vi "main.vi"() -> ()   [LabVIEW 2011]
uses:
  tab1.ctl
  System.Windows.Forms
  usb webcam list.ctl
  <vilib>/Instr/_visa.llb/VISA Configure Serial Port (Instr).vi
  <vilib>/vision/NI_Vision_Development_Module.lvlib
  <vilib>/Utility/file.llb/Read From Spreadsheet File (string).vi
  <vilib>/Utility/file.llb/Write To Spreadsheet File (string).vi
panel:
  out "height less than 1cm(80pixels)":bool
  out "image features":T1
  out "Vertical Profile":sgl[](graph)
  in  "cam on":bool=TRUE
  out "Clipboard has an image?":bool
  in  "stop for camera":bool
  in  "Select options":T2(radio)=enum."Database testing"
  in  "Tab Control 2":T3(tab)
  in  "Show cyl list":bool
  out "cust list":string[](array[string])
  in  "select cust":string
  out "cyl list":string[](array[string])
  out "cust data":string[][](array[string])
  out "weightage Array":u8[][](array[numeric])
  out "read matrix":u8[][](array[numeric])
  out "correlation":u8[](array[numeric])
  in  "Tab Control":T4
  in  "9600 8-N-1 none":u32=9600
  in  "COM port":refnum<visa-resource-name>
  in  "PictureBox":refnum<k24>(container)
  out "error initialising":bool
  in  "capture":bool
  in  "OK Button":bool
  in  "File Path":path
  in  "select source":enum32{"user selectable", "constant"}(radio)
  in  "Reject roi border particles":bool=TRUE
  in  "invert":bool
  in  "manual crop":bool
  in  "Erode process":bool
  in  "select char set source":enum32{"user selectable", "constant"}(ring)
  in  "File Path for char set":path
  in  "select DB source":enum32{"user selectable", "constant"}(ring)
  in  "DB Path in":path
  out "original image":T5(plugin-control)
  out "processed image":T5(plugin-control)
  out "array of mean":sgl[](array[numeric])
  out "Array of SD":sgl[](array[numeric])
  in  "OCRed output":T5(plugin-control)
  out "Read string (black objects)":string
  out "angle of rotation":dbl
  out "image rotated by :":dbl
  out "After Database Probability correction":string
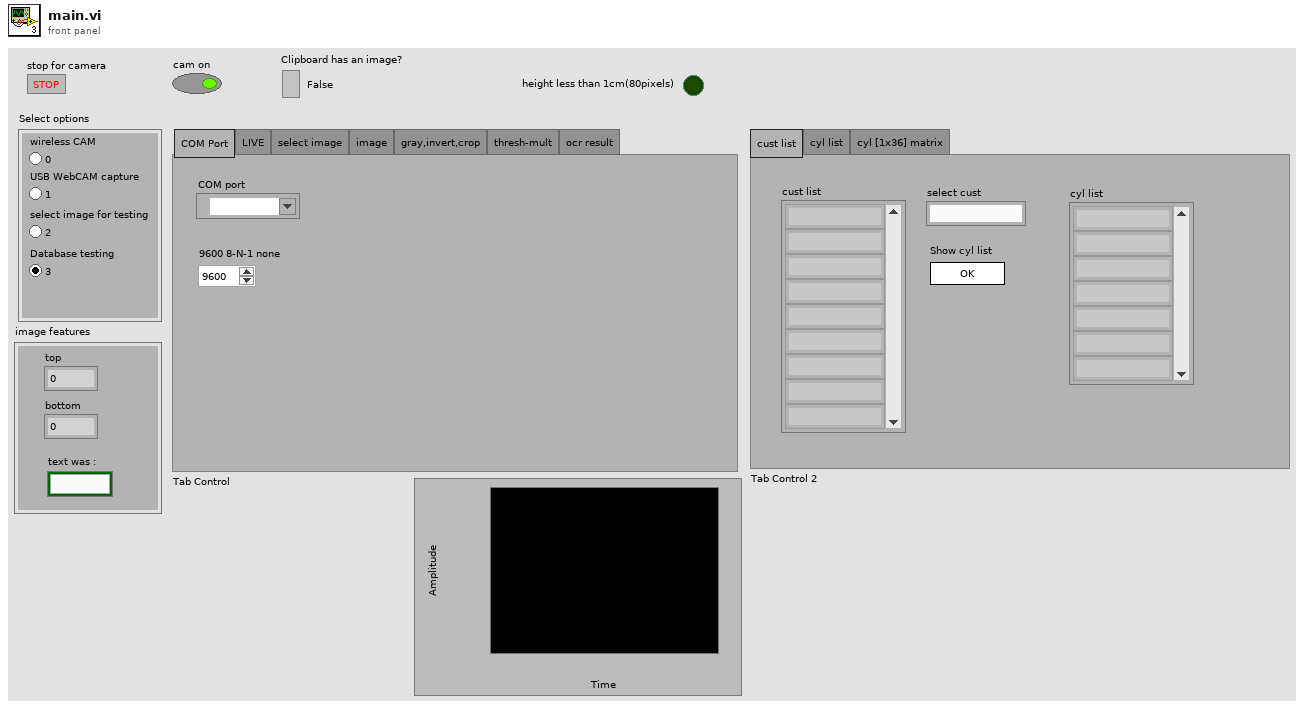
[diagram p1: front panel]
types:
  T1 = cluster{"text was :":bool, "top":i32, "bottom":i32}
  T2 = enum32{"wireless CAM", "USB WebCAM capture", "select image for testing", "Database testing"}
  T3 = enum32{"cust list", "cyl list", "cyl [1x36] matrix"}
  T4 = typedef "tab1.ctl" = enum32{"COM Port", "LIVE", "select image", "image", "gray,invert,crop", "thresh-mult", "ocr result"}
  T5 = typedef "IMAQ Image.ctl" = refnum<image>
  T6 = typedef "usb webcam list.ctl" = enum16{"floating controls", "Initialize", "capture", "processing image", "ocr unit", "close all sessions", "stop"}
  T7 = typedef "Image Type" = u32
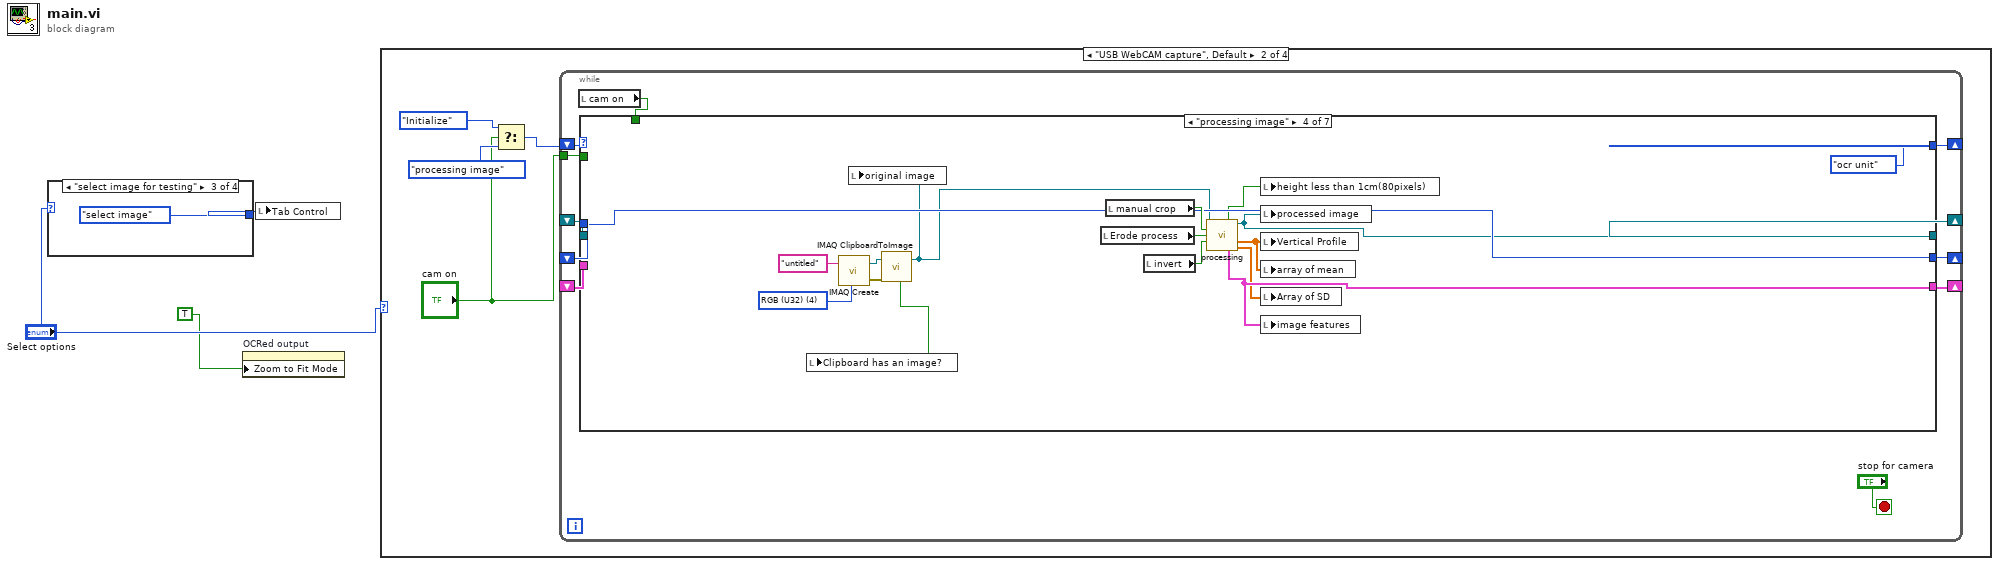
[diagram p0: block diagram]
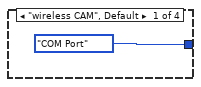
[diagram p2: hidden frame]
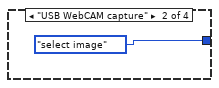
[diagram p3: hidden frame]
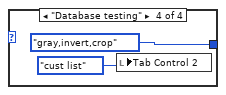
[diagram p4: hidden frame]
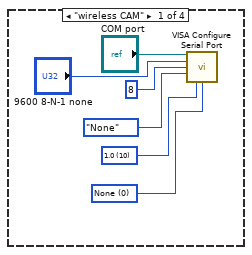
[diagram p5: hidden frame]
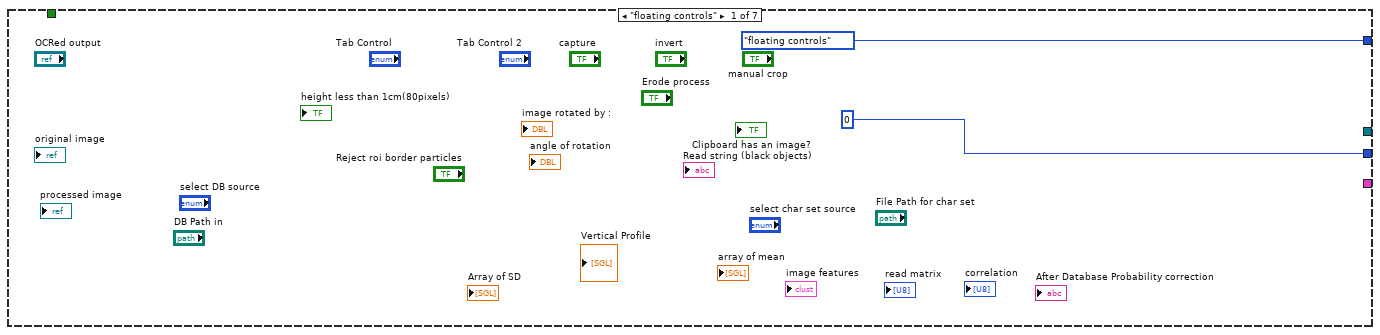
[diagram p6: hidden frame]
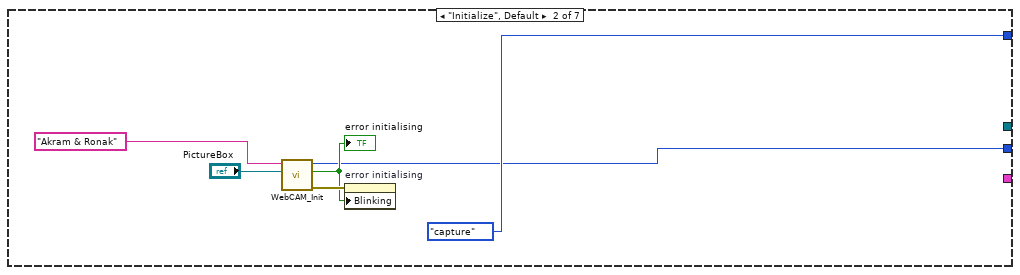
[diagram p7: hidden frame]
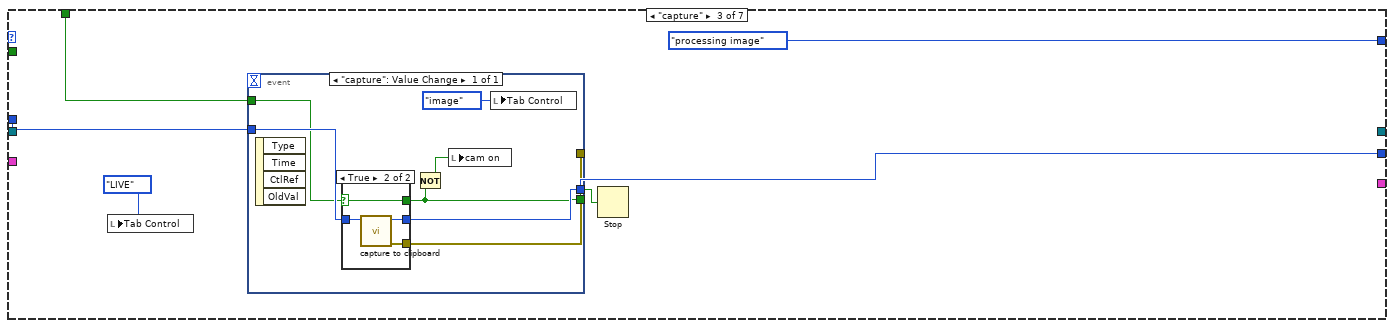
[diagram p8: hidden frame]
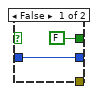
[diagram p9: hidden frame]
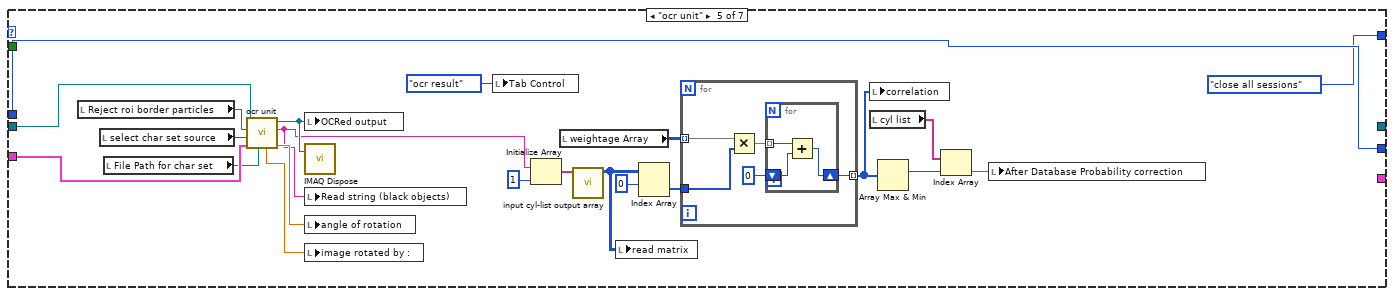
[diagram p10: hidden frame]
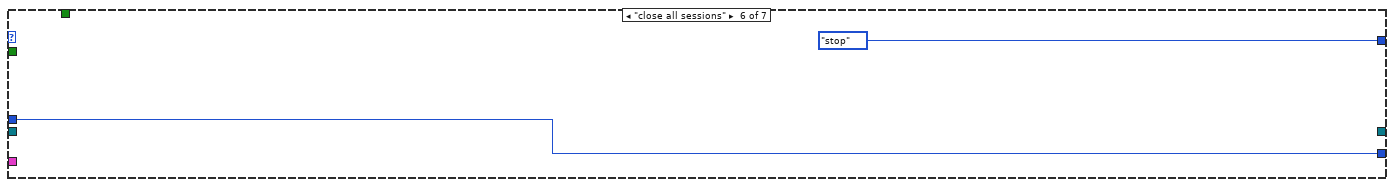
[diagram p11: hidden frame]
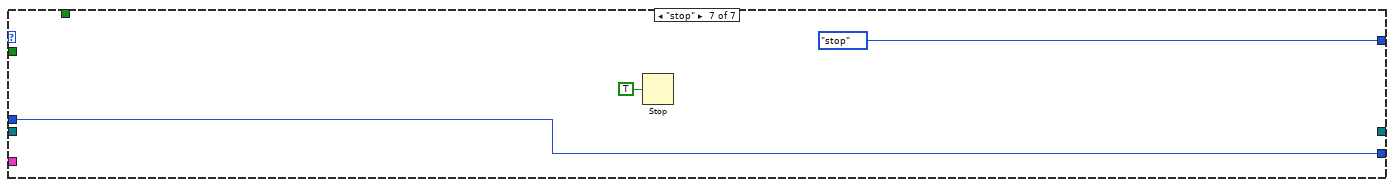
[diagram p12: hidden frame]
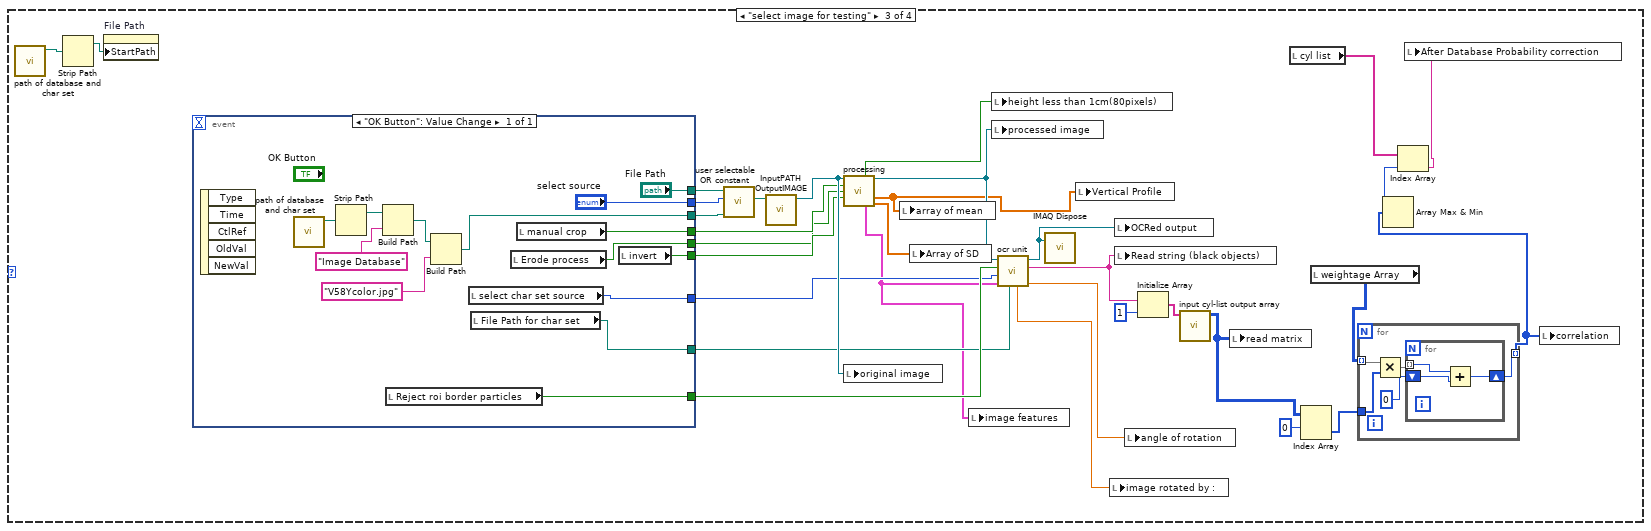
[diagram p13: hidden frame]
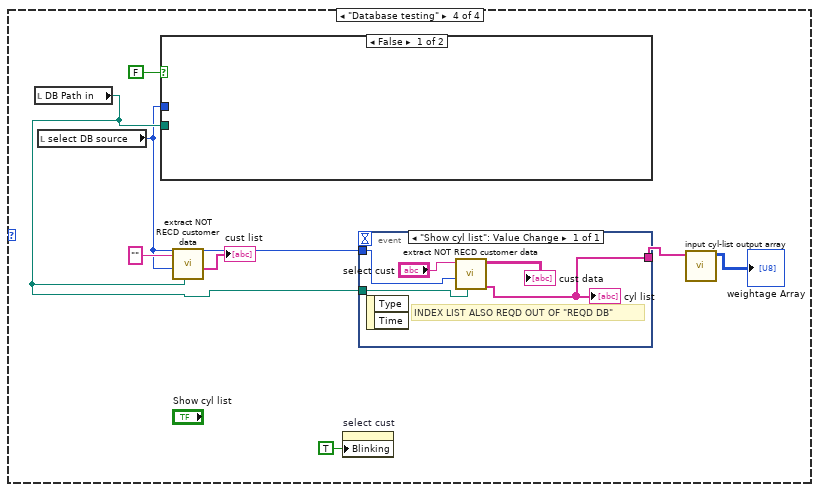
[diagram p14: hidden frame]
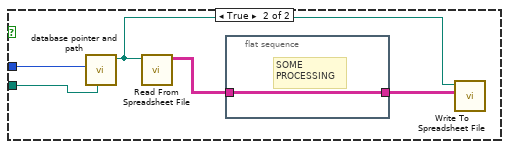
[diagram p15: hidden frame]
diagram:
  n1 = case shown="\"select image for testing\"" "Select options" {
    tunnel: [tab1."COM Port" ("Tab Control") tab1."select image" ("Tab Control") tab1."select image" ("Tab Control") tab1."gray,invert,crop" ("Tab Control")] -> w2
    frame "wireless CAM", Default {
    }
    frame "USB WebCAM capture" {
    }
    frame "select image for testing" {
    }
    frame "Database testing" {
      n2 = local write "Tab Control 2"(enum32{"cust list", "cyl list"}."cust list" ("Tab Control 2")) -> ()
    }
  }
  n3 = property on="OCRed output" class="ImageControl"("Zoom to Fit Mode"=TRUE) -> ()  [unwired: 2 in, 2 out]
  n4 = local write "Tab Control"(w2) -> ()
  n5 = case shown="\"USB WebCAM capture\", Default" "Select options" {
    frame "wireless CAM" {
      w10 = u16 10 items=["1.0"=10, "1.5"=15, "2.0"=20] ("stop bits (10: 1 bit)")
      w11 = u16 0 items=["None", "XON/XOFF", "RTS/CTS", "XON/XOFF & RTS/CTS", "DTR/DSR", "XON/XOFF & DTR/DSR"] ("flow control (0:none)")
      n6 = call-poly "VISA Configure Serial Port"("VISA resource name"="COM port", "baud rate (9600)"="9600 8-N-1 none", "data bits (8)"=u16 8, "parity (0:none)"=enum16{"None", "Odd", "Even", "Mark", "Space"}."None", "stop bits (10: 1 bit)"=w10, "flow control (0:none)"=w11) -> ()  [unwired: 8 in, 2 out]
    }
    frame "USB WebCAM capture", Default {
      n7 = Select(t=usb_webcam_list."Initialize" ("Beginning State"), s="cam on", f=usb_webcam_list."processing image" ("Beginning State")) -> (s? t:f=w17:T6)
      n8 = while {
        shift-right: [w27] -> _
        shift-left: w17 -> [w29]
        shift-right: [w28] -> _
        shift-left: _ -> [w26]
        shift-right: [w25] -> _
        shift-left: _ -> [w24]
        tunnel: "cam on" -> [w22]
        shift-right: [w20] -> _
        shift-left: _ -> [w19]
        stop <- "stop for camera" stop-if-true
        n9 = local read "cam on"() -> (w21:bool)
        n10 = case shown="\"processing image\"" w29 {
          tunnel: [u32 0 ("hwnd out") w32 w42 w70 w94 w104 w107] -> w28
          tunnel: [usb_webcam_list."floating controls" ("Beginning State") usb_webcam_list."capture" ("Beginning State") usb_webcam_list."processing image" ("Beginning State") usb_webcam_list."ocr unit" ("Beginning State") usb_webcam_list."close all sessions" ("Beginning State") usb_webcam_list."stop" ("Beginning State") usb_webcam_list."stop" ("Beginning State")] -> w27
          tunnel: w26 -> [_ _ w43 w70 w94 w104 w107]
          tunnel: [_ _ _ w63 _ _ _] -> w25
          tunnel: w24 -> [_ _ _ _ w93 _ _]
          tunnel: w22 -> [_ _ _ _ _ _ _]
          tunnel: w21 -> [_ _ w40 _ _ _ _]
          tunnel: [_ _ _ w67 _ _ _] -> w20
          tunnel: w19 -> [_ _ _ _ w89 _ _]
          frame "floating controls" {
          }
          frame "Initialize", Default {
            n11 = call "WebCAM_Init.vi"("PictureBox 2"="PictureBox", "Window Title"="Akram & Ronak") -> ("error out"=w35:errorcluster, "error initialising"=w34:bool, "hwnd"=w32:u32)  [unwired: 6 in, 1 out]
            "error initialising" <- w34
            n12 = property on="error initialising" class="Bool (strict)"(error in=w35, "Blinking"=w34) -> ()  [unwired: 1 in, 2 out]
          }
          frame "capture" {
            n13 = local write "Tab Control"(tab1."LIVE" ("Tab Control")) -> ()
            n14 = event shown="[0] \"capture\": Value Change" {
              selector: _ -> [_]
              dyn-events: _ -> [_]
              timeout: _ -> [_]
              tunnel: [w50] -> _
              tunnel: w43 -> [w49]
              tunnel: [w48] -> w42
              tunnel: w40 -> [w47]
              tunnel: [w45] -> w38
              event "capture": Value Change {
                n15 = event-data() -> ()  [unwired: 1 in, 4 out]
                n16 = case shown="True" w47 {
                  selector: w47 -> [_ w53]
                  tunnel: [_ w56] -> w50
                  tunnel: w49 -> [w52 w55]
                  tunnel: [w52 w54] -> w48
                  tunnel: [FALSE w53] -> w45
                  frame False {
                  }
                  frame True {
                    n17 = call "capture to clipboard.vi"("hwnd in"=w55) -> ("error out"=w56:errorcluster, "hwnd out"=w54:u32)  [unwired: 9 in]
                  }
                }
                n18 = Not(x=w45) -> (.not. x?=w44:bool)
                n19 = local write "cam on"(w44) -> ()
                n20 = local write "Tab Control"(tab1."image" ("Tab Control")) -> ()
              }
            }
            n21 = Stop(stop? (T)=w38) -> ()
          }
          frame "processing image" {
            w59 = T7 4 items=["Grayscale (U8)", "Grayscale (I16)", "Grayscale (SGL)", "Complex (CSG)", "RGB (U32)", "HSL (U32)", "RGB (U64)", "Grayscale (U16)"] ("Image Type")
            n22 = call "IMAQ Create"("Image Name"="untitled", "Image Type"=w59) -> ("New Image"=w60:T5, "error out"=w58:errorcluster)  [unwired: 2 in, 1 out]
            n23 = call "IMAQ ClipboardToImage"("error in (no error)"=w58, "Image"=w60) -> ("Clipboard has an image?"=w61:bool, "Image Out"=w57:T5)  [unwired: 3 in, 2 out]
            n24 = local write "Clipboard has an image?"(w61) -> ()
            n25 = local write "original image"(w57) -> ()
            n26 = local read "Erode process"() -> (w64:bool)
            n27 = local read "manual crop"() -> (w72:bool)
            n28 = local read "invert"() -> (w71:bool)
            n29 = call "processing.vi"("Refnum in"=w57, "manual crop"=w72, "Erode process"=w64, "invert"=w71) -> ("height less than 1cm(80pixels)"=w68:bool, "after complete processing"=w63:T5, "array of mean"=w65:sgl[], "image features"=w67:T1, "Array of SD"=w66:sgl[])  [unwired: 7 in]
            n30 = local write "height less than 1cm(80pixels)"(w68) -> ()
            n31 = local write "processed image"(w63) -> ()
            n32 = local write "Vertical Profile"(w65) -> ()
            n33 = local write "array of mean"(w65) -> ()
            n34 = local write "Array of SD"(w66) -> ()
            n35 = local write "image features"(w67) -> ()
          }
          frame "ocr unit" {
            n36 = local read "Reject roi border particles"() -> (w91:bool)
            n37 = local read "select char set source"() -> (w88:enum32{"user selectable", "constant"})
            n38 = local read "File Path for char set"() -> (w87:path)
            n39 = call "ocr unit.vi"("File Path in"=w87, "image features"=w89, "select source"=w88, "reject roi border particles"=w91, "Refnum in"=w93) -> ("angle of rotation"=w76:dbl, "Read String"=w75:string, "Refnum out"=w92:T5, "image rotated by :"=w77:dbl)  [unwired: 2 in, 1 out]
            n40 = local write "OCRed output"(w92) -> ()
            n41 = call "IMAQ Dispose"("Image"=w92) -> ()  [unwired: 2 in, 4 out]
            n42 = local write "Read string (black objects)"(w75) -> ()
            n43 = local write "angle of rotation"(w76) -> ()
            n44 = local write "image rotated by :"(w77) -> ()
            n45 = local write "Tab Control"(tab1."ocr result" ("Tab Control")) -> ()
            n46 = Initialize Array(w75, 1 ("dimension size")) -> (w81:string[])
            n47 = local read "weightage Array"() -> (w83:u8[][])
            n48 = call "input cyl-list output array.vi"("cyl list"=w81) -> ("Array"=w82:u8[][])  [unwired: 10 in]
            n49 = local write "read matrix"(w82) -> ()
            n50 = Index Array(array=w82, index (row)=0) -> (element=w78:u8[])  [unwired: 1 in]
            n51 = for {
              tunnel: w78 -> [w98]
              tunnel: w83 -> [w99] mode=indexing
              tunnel: [w95] -> w74 mode=indexing
              n52 = Multiply(x=w99, y=w98) -> (x*y=w97:u8[])
              n53 = for {
                tunnel: w97 -> [w102] mode=indexing
                shift-right: [w101] -> w95
                shift-left: u8 0 -> [w100]
                n54 = Add(x=w102, y=w100) -> (x+y=w101:u8)
              }
            }
            n55 = local write "correlation"(w74) -> ()
            n56 = local read "cyl list"() -> (w84:string[])
            n57 = Array Max & Min(array=w74) -> (max index (indices)=w85:i32)  [unwired: 3 out]
            n58 = Index Array(array=w84, index=w85) -> (element=w86:string)
            n59 = local write "After Database Probability correction"(w86) -> ()
          }
          frame "close all sessions" {
          }
          frame "stop" {
            n60 = Stop(stop? (T)=TRUE) -> ()
          }
        }
      }
    }
    frame "select image for testing" {
      n61 = call "path of database and char set.vi"() -> ("appended path"=w139:path)  [unwired: 11 in]
      n62 = Strip Path(path=w139) -> (stripped path=w114:path)  [unwired: 1 out]
      n63 = property on="File Path" class="Path"("StartPath"=w114) -> ()  [unwired: 2 in, 2 out]
      n64 = event shown="[0] \"OK Button\": Value Change" {
        selector: _ -> [_]
        dyn-events: _ -> [_]
        timeout: _ -> [_]
        tunnel: ["File Path"] -> w110
        tunnel: ["select source"] -> w109
        tunnel: [w151] -> w135
        tunnel: [w150] -> w134
        tunnel: [w149] -> w133
        tunnel: [w148] -> w132
        tunnel: [w146] -> w108
        tunnel: [w145] -> w122
        tunnel: [w144] -> w121
        event "OK Button": Value Change {
          n65 = event-data() -> ()  [unwired: 1 in, 5 out]
          n66 = call "path of database and char set.vi"() -> ("appended path"=w143:path)  [unwired: 11 in]
          n67 = Strip Path(path=w143) -> (stripped path=w142:path)  [unwired: 1 out]
          n68 = Build Path(base path=w142, name or relative path="Image Database") -> (appended path=w141:path)
          n69 = local read "Reject roi border particles"() -> (w149:bool)
          n70 = Build Path(base path=w141, name or relative path="V58Ycolor.jpg") -> (appended path=w146:path)
          n71 = local read "select char set source"() -> (w145:enum32{"user selectable", "constant"})
          n72 = local read "File Path for char set"() -> (w144:path)
          n73 = local read "Erode process"() -> (w148:bool)
          n74 = local read "manual crop"() -> (w151:bool)
          n75 = local read "invert"() -> (w150:bool)
        }
      }
      n76 = call "user selectable OR constant.vi"("Constant Path in"=w108, "select source"=w109, "File Path in"=w110) -> ("appended path"=w111:path)  [unwired: 8 in]
      n77 = call "InputPATH   OutputIMAGE.vi"("appended path"=w111) -> ("Refnum out"=w137:T5)  [unwired: 9 in, 1 out]
      n78 = call "processing.vi"("Refnum in"=w137, "manual crop"=w135, "Erode process"=w132, "invert"=w134) -> ("height less than 1cm(80pixels)"=w131:bool, "after complete processing"=w136:T5, "array of mean"=w115:sgl[], "image features"=w117:T1, "Array of SD"=w116:sgl[])  [unwired: 7 in]
      n79 = local write "original image"(w137) -> ()
      n80 = local write "array of mean"(w115) -> ()
      n81 = local write "Array of SD"(w116) -> ()
      n82 = local write "image features"(w117) -> ()
      n83 = local write "height less than 1cm(80pixels)"(w131) -> ()
      n84 = local write "processed image"(w136) -> ()
      n85 = call "ocr unit.vi"("File Path in"=w121, "image features"=w117, "select source"=w122, "reject roi border particles"=w133, "Refnum in"=w136) -> ("angle of rotation"=w113:dbl, "Read String"=w129:string, "Refnum out"=w138:T5, "image rotated by :"=w112:dbl)  [unwired: 2 in, 1 out]
      n86 = call "IMAQ Dispose"("Image"=w138) -> ()  [unwired: 2 in, 4 out]
      n87 = local write "Vertical Profile"(w115) -> ()
      n88 = local write "image rotated by :"(w112) -> ()
      n89 = local write "OCRed output"(w138) -> ()
      n90 = local write "Read string (black objects)"(w129) -> ()
      n91 = local write "angle of rotation"(w113) -> ()
      n92 = Initialize Array(w129, 1 ("dimension size")) -> (w130:string[])
      n93 = call "input cyl-list output array.vi"("cyl list"=w130) -> ("Array"=w118:u8[][])  [unwired: 10 in]
      n94 = local write "read matrix"(w118) -> ()
      n95 = local read "cyl list"() -> (w123:string[])
      n96 = Index Array(array=w118, index (row)=0) -> (element=w127:u8[])  [unwired: 1 in]
      n97 = local read "weightage Array"() -> (w125:u8[][])
      n98 = for {
        tunnel: w127 -> [w157]
        tunnel: w125 -> [w158] mode=indexing
        tunnel: [w154] -> w119 mode=indexing
        n99 = Multiply(x=w158, y=w157) -> (x*y=w156:u8[])
        n100 = for {
          tunnel: w156 -> [w161] mode=indexing
          shift-right: [w160] -> w154
          shift-left: u8 0 -> [w159]
          n101 = Add(x=w161, y=w159) -> (x+y=w160:u8)
        }
      }
      n102 = Array Max & Min(array=w119) -> (max index (indices)=w124:i32)  [unwired: 3 out]
      n103 = Index Array(array=w123, index=w124) -> (element=w120:string)
      n104 = local write "After Database Probability correction"(w120) -> ()
      n105 = local write "correlation"(w119) -> ()
    }
    frame "Database testing" {
      n106 = local read "DB Path in"() -> (w163:path)
      n107 = local read "select DB source"() -> (w162:enum32{"user selectable", "constant"})
      n108 = case shown="False" FALSE {
        tunnel: w162 -> [_ w176]
        tunnel: w163 -> [_ w175]
        frame False {
        }
        frame True {
          n109 = call "database pointer and path.vi"("File Path in"=w175, "select source"=w176) -> ("appended path"=w178:path)  [unwired: 8 in, 1 out]
          n110 = call-poly <vilib>:"Read From Spreadsheet File.vi"("file path (dialog if empty)"=w178) -> ("all rows"=w179:string[][])  [unwired: 6 in, 4 out]
          n111 = flat-sequence {
            tunnel: w179 -> [w180]
            tunnel: [w180] -> w177
            frame #0 {
              # "SOME\nPROCESSING"
            }
          }
          n112 = call-poly <vilib>:"Write To Spreadsheet File.vi"("2D data"=w177, "file path (dialog if empty)"=w178) -> ()  [unwired: 6 in, 1 out]
        }
      }
      n113 = call "extract NOT RECD customer data.vi"("File Path in"=w163, "select source"=w162, "select cust"="") -> ("cust list"=→"cust list":string[])  [unwired: 6 in, 2 out]
      n114 = property on="select cust" class="Str"("Blinking"=TRUE) -> ()  [unwired: 2 in, 2 out]
      n115 = event shown="[0] \"Show cyl list\": Value Change" {
        selector: _ -> [_]
        dyn-events: _ -> [_]
        timeout: _ -> [_]
        tunnel: [w172] -> w165
        tunnel: w163 -> [w171]
        tunnel: w162 -> [w170]
        event "Show cyl list": Value Change {
          # "INDEX LIST ALSO REQD OUT OF \"REQD DB\""
          n116 = event-data() -> ()  [unwired: 1 in, 2 out]
          n117 = call "extract NOT RECD customer data.vi"("File Path in"=w171, "select source"=w170, "select cust"="select cust") -> ("cyl list"=w172:string[], "cust data"=→"cust data":string[][])  [unwired: 6 in, 1 out]
          "cyl list" <- w172
        }
      }
      n118 = call "input cyl-list output array.vi"("cyl list"=w165) -> ("Array"=→"weightage Array":u8[][])  [unwired: 10 in]
    }
  }
